vi "list - get file names - meta.vi"(5 "extension filter":string="*.dat", 6 "match index":i32=-1, 7 "regular expression":string="\\s*([0-9]+_.*?)\\.dat\\s*", 11 "folder path":path) -> (0 "full name Array":string[](array[string]), 1 "match Array":string[](array[string]), 2 "OK":bool)   [LabVIEW 2012]
uses:
  <vilib>/regexp/Match Regular Expression.xnode
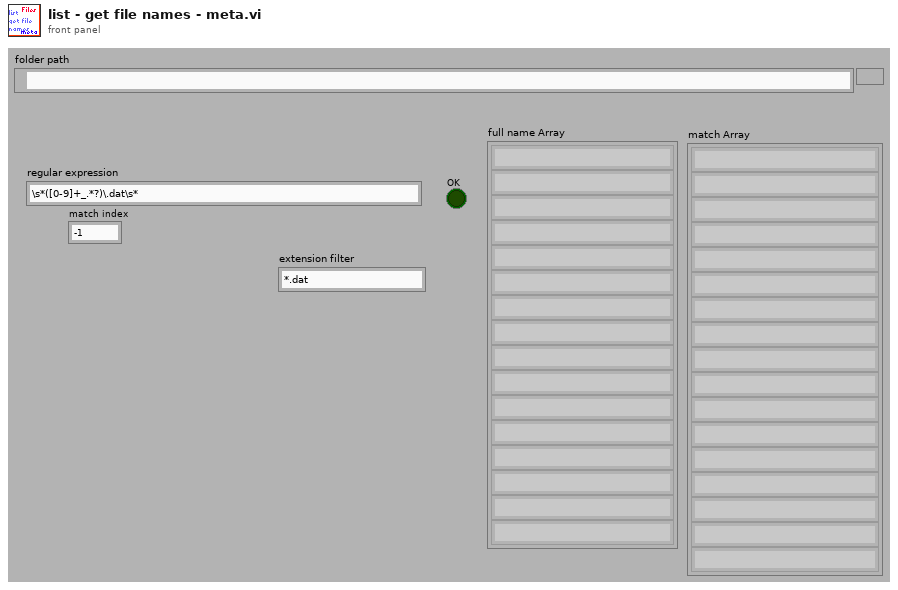
[diagram p1: front panel]
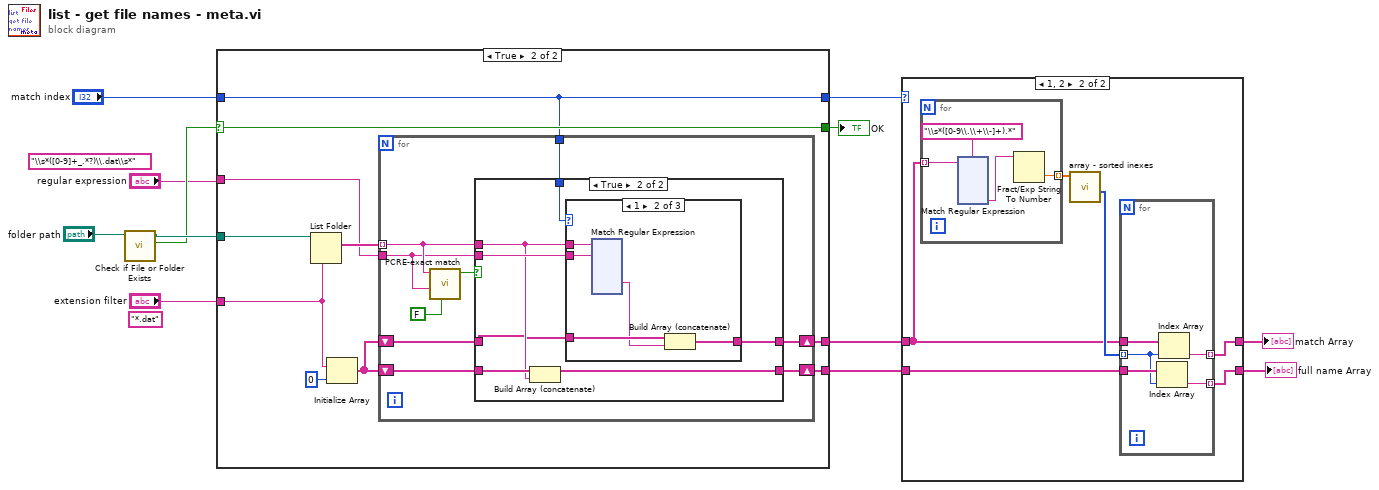
[diagram p0: block diagram]
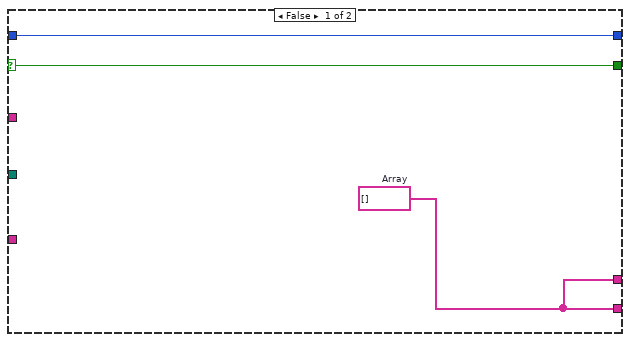
[diagram p3: hidden frame]
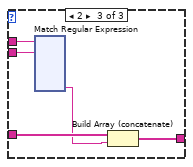
[diagram p6: hidden frame]
diagram:
  (unwired) "\\s*([0-9]+_.*?)\\.dat\\s*" ("regular expression")
  (unwired) "*.dat" ("pattern")
  n1 = call <vilib>:"Check if File or Folder Exists.vi"("path"="folder path") -> ("file or folder exists?"=w10:bool, "dup path"=w11:path)  [unwired: 8 in, 1 out]
  n2 = case shown="True" w10 {
    selector: w10 -> [w15 w19]
    tunnel: "extension filter" -> [_ w24]
    tunnel: "regular expression" -> [_ w22]
    tunnel: w11 -> [_ w21]
    tunnel: [w14 w20] -> w3
    tunnel: [w15 w19] -> w7
    tunnel: "match index" -> [w13 w16]
    tunnel: [w14 w18] -> w4
    tunnel: [w13 w16] -> w5
    frame False {
      w14 = string[] []  # Array
    }
    frame True {
      n3 = List Folder(path=w21, pattern=w24) -> (filenames=w25:string[])  [unwired: 2 in, 3 out]
      n4 = Initialize Array(w24, 0 ("dimension size")) -> (w17:string[])
      n5 = for {
        tunnel: w25 -> [w32] mode=indexing
        shift-right: [w33] -> w20
        shift-left: w17 -> [w34]
        tunnel: w22 -> [w30]
        tunnel: w16 -> [w28]
        shift-right: [w27] -> w18
        shift-left: w17 -> [w26]
        n6 = call "PCRE-exact match.vi"("quote specials"=FALSE ("Boolean"), "regular expression"=w30, "input string"=w32) -> ("exact match"=w31:bool)  [unwired: 7 in, 1 out]
        n7 = case shown="True" w31 {
          tunnel: w30 -> [_ w43]
          tunnel: w34 -> [w36 w42]
          tunnel: [w36 w41] -> w33
          tunnel: w32 -> [_ w40]
          tunnel: w28 -> [_ w39]
          tunnel: [w35 w38] -> w27
          tunnel: w26 -> [w35 w37]
          frame False {
          }
          frame True {
            n8 = Build Array (concatenate)(w42, w40) -> (w41:string[])
            n9 = case shown="1" w39 {
              tunnel: w43 -> [_ w49 w168]
              tunnel: w40 -> [_ w48 w167]
              tunnel: [w44 w47 w166] -> w38
              tunnel: w37 -> [w44 w46 w165]
              frame 0, Default {
              }
              frame 1 {
                n10 = xnode "Match Regular Expression"("input string"=w48, "regular expression"=w49) -> ("submatch 1"=w45:string)  [unwired: 4 in, 6 out]
                n11 = Build Array (concatenate)(w46, w45) -> (w47:string[])
              }
              frame 2 {
                n12 = xnode "Match Regular Expression"("input string"=w167, "regular expression"=w168) -> ("submatch 2"=w164:string)  [unwired: 4 in, 6 out]
                n13 = Build Array (concatenate)(w165, w164) -> (w166:string[])
              }
            }
          }
        }
      }
    }
  }
  "OK" <- w7
  n14 = case shown="1, 2" w5 {
    tunnel: w4 -> [w284 w288]
    tunnel: w3 -> [w283 w287]
    tunnel: [w284 w286] -> w2
    tunnel: [w283 w285] -> w1
    frame -1, Default {
    }
    frame 1, 2 {
      n15 = for {
        tunnel: w288 -> [w299] mode=indexing
        tunnel: [w296] -> w290 mode=indexing
        n16 = xnode "Match Regular Expression"("input string"=w299, "regular expression"="\\s*([0-9\\.\\+\\-]+).*") -> ("submatch 1"=w297:string)  [unwired: 4 in, 5 out]
        n17 = Fract/Exp String To Number(string=w297) -> (number=w296:dbl)  [unwired: 3 in, 1 out]
      }
      n18 = call "array - sorted inexes.vi"("x"=w290) -> ("index array"=w289:i32[])  [unwired: 9 in, 1 out]
      n19 = for {
        tunnel: w289 -> [w292] mode=indexing
        tunnel: w288 -> [w295]
        tunnel: [w294] -> w286 mode=indexing
        tunnel: w287 -> [w293]
        tunnel: [w291] -> w285 mode=indexing
        n20 = Index Array(array=w293, index=w292) -> (element=w291:string)
        n21 = Index Array(array=w295, index=w292) -> (element=w294:string)
      }
    }
  }
  "full name Array" <- w1
  "match Array" <- w2
